vi "SDCP BTR Test - Scope Mode.vi"() -> ()   [LabVIEW 2020]
uses:
  Typedefs/SDCP BTR Params.ctl
  Typedefs/SDCP - Serial Port Control - Commands.ctl
panel:
  out "Status":T1
  out "Time interval (ms)":u32[](array[numeric])
  in  "Number of tries":i32
  in  "Parameter IDs":u8[](array[numeric])=[8, 9, 10, 11]
  in  "Number of transfers":u16=1
  in  "Stop application":bool
  in  "Block transfer parameters file path":path=path "E:/Projects/System Diagnostics and Control Protocol/SDCP_LabVIEW/Parameter Files/test.btp"
  in  "VISA resource name":refnum<visa-resource-name>="COM5"
  in  "Baud rate":u32=115200
  # "Block transfer settings"
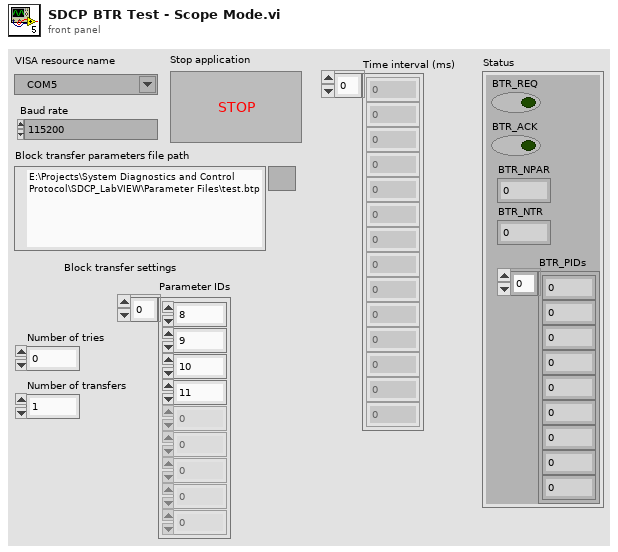
[diagram p1: front panel]
types:
  T1 = typedef "SDCP BTR Params.ctl" = cluster{"BTR_REQ":bool, "BTR_ACK":bool, "BTR_NPAR":i32, "BTR_NTR":i32, "BTR_PIDs":u8[]}
  T2 = typedef "SDCP - Serial Port Control - Commands.ctl" = enum16{"Open", "Read", "Write", "Get instance", "Close"}
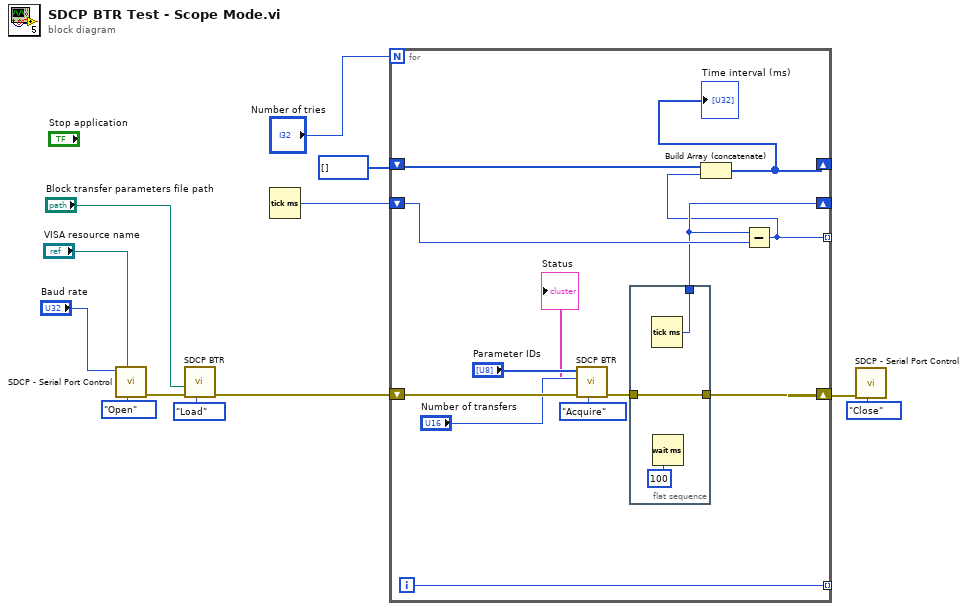
[diagram p0: block diagram]
diagram:
  n1 = call "SDCP - Serial Port Control.vi"("Command"=SDCP_-_Serial_Port_Control_-_Commands."Open", "VISA resource name"="VISA resource name", "Baud rate"="Baud rate") -> ("error out"=w12:errorcluster)  [unwired: 6 in, 2 out]
  n2 = call "SDCP BTR.vi"("Command"=enum16{"Load", "Acquire"}."Load", "error in (no error)"=w12, "Block transfer parameters file path"="Block transfer parameters file path") -> ("error out"=w6:errorcluster)  [unwired: 5 in, 3 out]
  n3 = Tick Count (ms)() -> (millisecond timer value=w2:u32)
  n4 = for {
    N: "Number of tries" -> [_]
    shift-right: [w19] -> w5
    shift-left: w6 -> [w25]
    shift-right: [w18] -> _
    shift-left: w2 -> [w21]
    tunnel: [w15] -> _ mode=indexing
    tunnel: [w17] -> _ mode=indexing
    shift-right: [w14] -> _
    shift-left: u32[] [] -> [w16]
    i -> [w17]
    n5 = call "SDCP BTR.vi"("Command"=enum16{"Load", "Acquire"}."Acquire", "error in (no error)"=w25, "Number of transfers"="Number of transfers", "Parameter IDs"="Parameter IDs") -> ("error out"=w20:errorcluster, "Status"=→"Status":T1)  [unwired: 4 in, 2 out]
    n6 = flat-sequence {
      tunnel: w20 -> [w28]
      tunnel: [w28] -> w19
      tunnel: [w26] -> w18
      frame #0 {
        n7 = Tick Count (ms)() -> (millisecond timer value=w26:u32)
        n8 = Wait (ms)(milliseconds to wait=u32 100) -> ()  [unwired: 1 out]
      }
    }
    n9 = Subtract(x=w18, y=w21) -> (x-y=w15:u32)
    n10 = Build Array (concatenate)(w16, w15) -> (w14:u32[])
    "Time interval (ms)" <- w14
  }
  n11 = call "SDCP - Serial Port Control.vi"("Command"=SDCP_-_Serial_Port_Control_-_Commands."Close", "error in (no error)"=w5) -> ()  [unwired: 7 in, 3 out]
